vi "Defer Panel Updates (Init).vi"(6 "Controls":refnum<vi>[](array[refnum]), 8 "error in (no error)":errorcluster, 10 "Defer Panel Updates? [T]":bool=TRUE, 11 "Registry Control Reference Accessor in":refnum<class "Registry Ctrl Ref Accessor.lvclass">) -> (0 "error out":errorcluster, 3 "Registry Control Reference Accessor out":refnum<class "Registry Ctrl Ref Accessor.lvclass">, 4 "Panel refs":refnum<vi>[](array[refnum]))   [LabVIEW 2013, in "Registry Ctrl Ref Accessor.lvclass"]
doc: "Copyright 2018, Carya Automatisering, Wiebe Walstra."
uses:
  Registry Ctrl Ref Accessor.lvclass
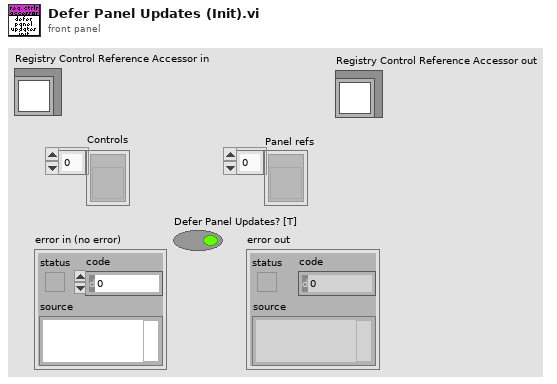
[diagram p1: front panel]
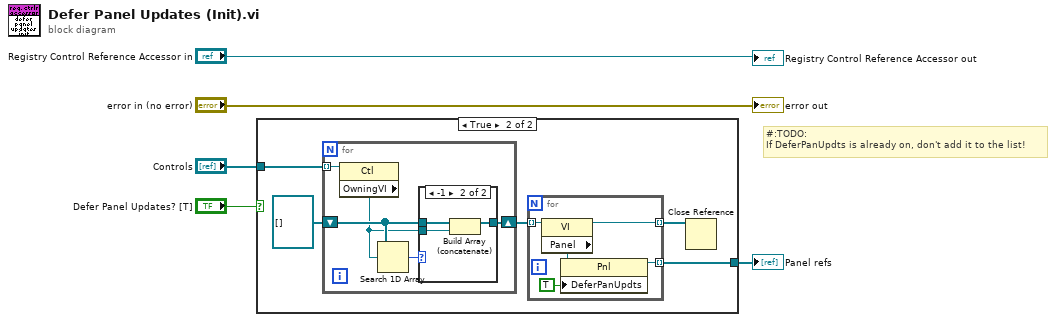
[diagram p0: block diagram]
diagram:
  # "#:TODO:\nIf DeferPanUpdts is already on, don't add it to the list!"
  n1 = case shown="True" "Defer Panel Updates? [T]" {
    tunnel: "Controls" -> [_ w10]
    tunnel: [_ w7] -> w2
    frame False {
    }
    frame True {
      n2 = for {
        tunnel: w10 -> [w20] mode=indexing
        shift-right: [w17] -> w8
        shift-left: refnum<vi>[] [] -> [w19]
        n3 = property class="Ctl"(reference=w20) -> ("OwningVI"=w18:refnum<vi>)  [unwired: 1 in, 2 out]
        n4 = Search 1D Array(1D array=w19, element=w18) -> (index of element=w16:i32)  [unwired: 1 in]
        n5 = case shown="-1" w16 {
          tunnel: w19 -> [w21 w24]
          tunnel: w18 -> [_ w23]
          tunnel: [w21 w22] -> w17
          frame Default {
          }
          frame -1 {
            n6 = Build Array (concatenate)(w24, w23) -> (w22:refnum<vi>[])
          }
        }
      }
      n7 = for {
        tunnel: w8 -> [w15] mode=indexing
        tunnel: [w12] -> w7 mode=indexing
        tunnel: [w11] -> w6 mode=indexing
        n8 = property class="VI"(reference=w15) -> (reference out=w11:refnum<vi>, "Panel"=w14:refnum<vi>)  [unwired: 1 in, 1 out]
        n9 = property class="Pnl"(reference=w14, "DeferPanUpdts"=TRUE ("Defer Panel Updates")) -> (reference out=w12:refnum<vi>)  [unwired: 1 in, 1 out]
      }
      n10 = Close Reference(reference=w6) -> ()  [unwired: 1 in, 1 out]
    }
  }
  "Panel refs" <- w2
  "error out" <- "error in (no error)"
  "Registry Control Reference Accessor out" <- "Registry Control Reference Accessor in"
